vi "Create Session.vi"(5 "Session in":refnum<class "Session.lvclass">, 7 "Close Session":refnum<user-event>, 8 "error in (no error)":errorcluster, 9 "Request":refnum<queue>, 10 "Keep Alive (s)":i32, 11 "Connection":refnum<class "Connection.lvclass">) -> (0 "error out":errorcluster, 3 "Session":refnum<class "Session.lvclass">)   [LabVIEW 2013, in "MQTT Base.lvlib" / "Session.lvclass"]
uses:
  Session.lvclass
  MQTT_Connection/Connection/Connection.lvclass
  Base Class/Request -- cluster.ctl
  <vilib>/LabVIEW Open Source Project/MQTT Control Packets/Control Packets/ControlPacket/ControlPacket.lvclass
  Base Class/Response -- cluster.ctl
  Session State -- cluster.ctl
  <vilib>/LabVIEW Open Source Project/MQTT Control Packets/Control Packets/SUBSCRIBE/Topic Subscription -- cluster.ctl
  <vilib>/LabVIEW Open Source Project/MQTT Control Packets/Control Packets/ControlPacket/QualityOfService -- enum.ctl
  <vilib>/LabVIEW Open Source Project/MQTT Control Packets/Control Packets/ControlPacket/Pending Transmission -- cluster.ctl
  Pending ACKs -- cluster.ctl
  Session.lvclass/Session.ctl
  Base Class/MQTT_Base.lvclass
  <vilib>/LabVIEW Open Source Project/MQTT Control Packets/Control Packets/SUBSCRIBE/SUBSCRIBE.lvclass
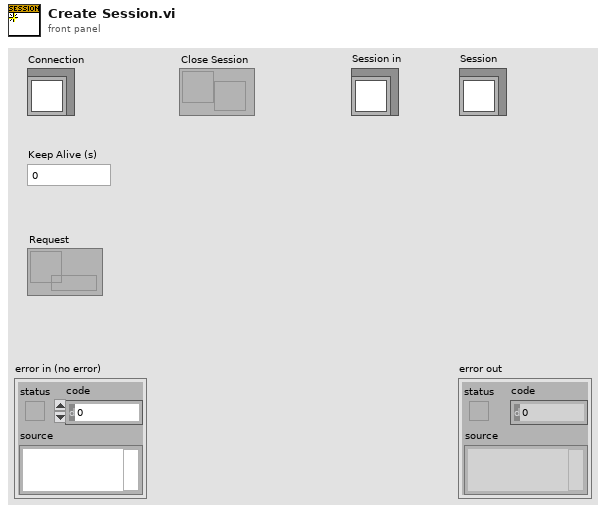
[diagram p1: front panel]
types:
  T1 = typedef "MQTT Base.lvlib/MQTT_Base.lvclass/Response -- cluster.ctl" = cluster{"Packet":refnum<class "ControlPacket.lvclass">, "Protocol Error":errorcluster, "disconnect session":bool, "[ACK]":refnum<notifier>[]}
  T2 = typedef "MQTT Base.lvlib/Session.lvclass/Session State -- cluster.ctl" = cluster{"CleanSession":bool, "Client ID":string, "Subscriptions":T3[], "Pending Transmissions":T5[], "Pending ACKs":T6[]}
  T3 = typedef "MQTT_Control_Packets.lvlib/SUBSCRIBE.lvclass/Topic Subscription -- cluster.ctl" = cluster{"Topic Filter":string, "QoS":T4}
  T4 = typedef "MQTT_Control_Packets.lvlib/ControlPacket.lvclass/QualityOfService -- enum.ctl" = enum16{"0 (At Most Once)", "1 (At Least Once)", "2 (Exactly Once)"}
  T5 = typedef "MQTT_Control_Packets.lvlib/ControlPacket.lvclass/Pending Transmission -- cluster.ctl" = cluster{"Message":refnum<class "ControlPacket.lvclass">, "QoS":T4, "Tx-Rx":bool}
  T6 = typedef "MQTT Base.lvlib/Session.lvclass/Pending ACKs -- cluster.ctl" = cluster{"Message":refnum<class "ControlPacket.lvclass">, "[ACK]":refnum<notifier>[], "Packet Identifier":u16}
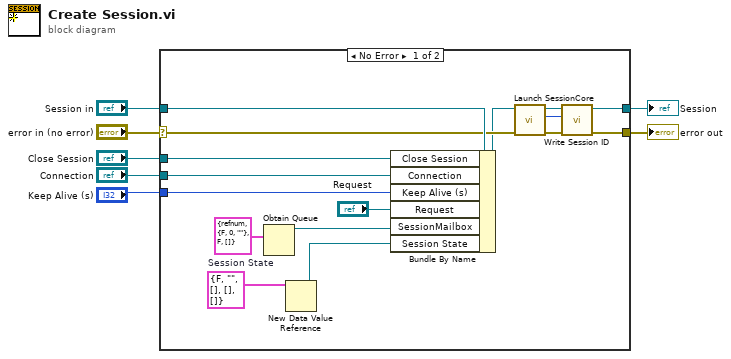
[diagram p0: block diagram]
diagram:
  n1 = case shown="No Error" "error in (no error)" {
    selector: "error in (no error)" -> [w16 w24]
    tunnel: [w9 w24] -> w6
    tunnel: [w15 w23] -> w4
    tunnel: "Session in" -> [w21 w23]
    tunnel: "Keep Alive (s)" -> [w19 _]
    tunnel: "Connection" -> [w18 _]
    tunnel: "Close Session" -> [w14 _]
    frame No Error {
      w13 = T2 {"CleanSession"=FALSE, "Client ID"="", "Subscriptions"=[], "Pending Transmissions"=[], "Pending ACKs"=[]}  # Session State
      n2 = Obtain Queue(element data type=T1 {"Packet"=refnum, "Protocol Error"={"status"=FALSE, "code"=0, "source"=""}, "disconnect session"=FALSE, "[ACK]"=[]} ("Response")) -> (queue out=w22:refnum<queue>)  [unwired: 4 in, 2 out]
      n3 = New Data Value Reference(data value=w13) -> (data value reference=w12:refnum<data-value>)  [unwired: 1 in, 1 out]
      n4 = Bundle By Name(cluster=w21, "Close Session"=w14, "Connection"=w18, "Keep Alive (s)"=w19, "Request"="Request", "SessionMailbox"=w22, "Session State"=w12) -> (w8:refnum<class "Session.lvclass">)
      n5 = call "Launch SessionCore.vi"("error in (no error)"=w16, "Session in"=w8) -> ("error out"=w9:errorcluster, "Session ID"=w11:i32, "Session out"=w10:refnum<class "Session.lvclass">)  [unwired: 7 in]
      n6 = call "Write Session ID.vi"("Session ID"=w11, "Session in"=w10) -> ("Session out"=w15:refnum<class "Session.lvclass">)  [unwired: 8 in, 1 out]
    }
    frame Error {
    }
  }
  "error out" <- w6
  "Session" <- w4
